vi "MGCC_FntStaMach_Flag_auto.vi"() -> (0 "Array":bool[](array[boolean]))   [LabVIEW 2016]
uses:
  Abnormal Fault State Control/Sub_VIs/Fault_Abnormal_state.vi
  Unplanned islanding (He Yin)/Sub Vis/UnplanISD_Global.vi
panel:
  in  "Feeder #2 energized":bool
  in  "Feeder #1 energized":bool
  in  "PCC_5 IR position":bool
  in  "PCC_4 IR position":bool
  in  "Feeder #5 energized":bool
  in  "Feeder #4 energized":bool
  in  "Feeder #3 energized":bool
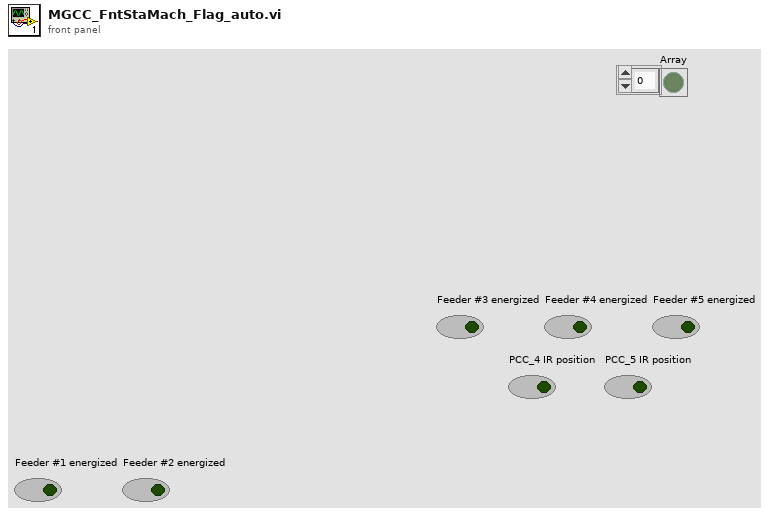
[diagram p1: front panel]
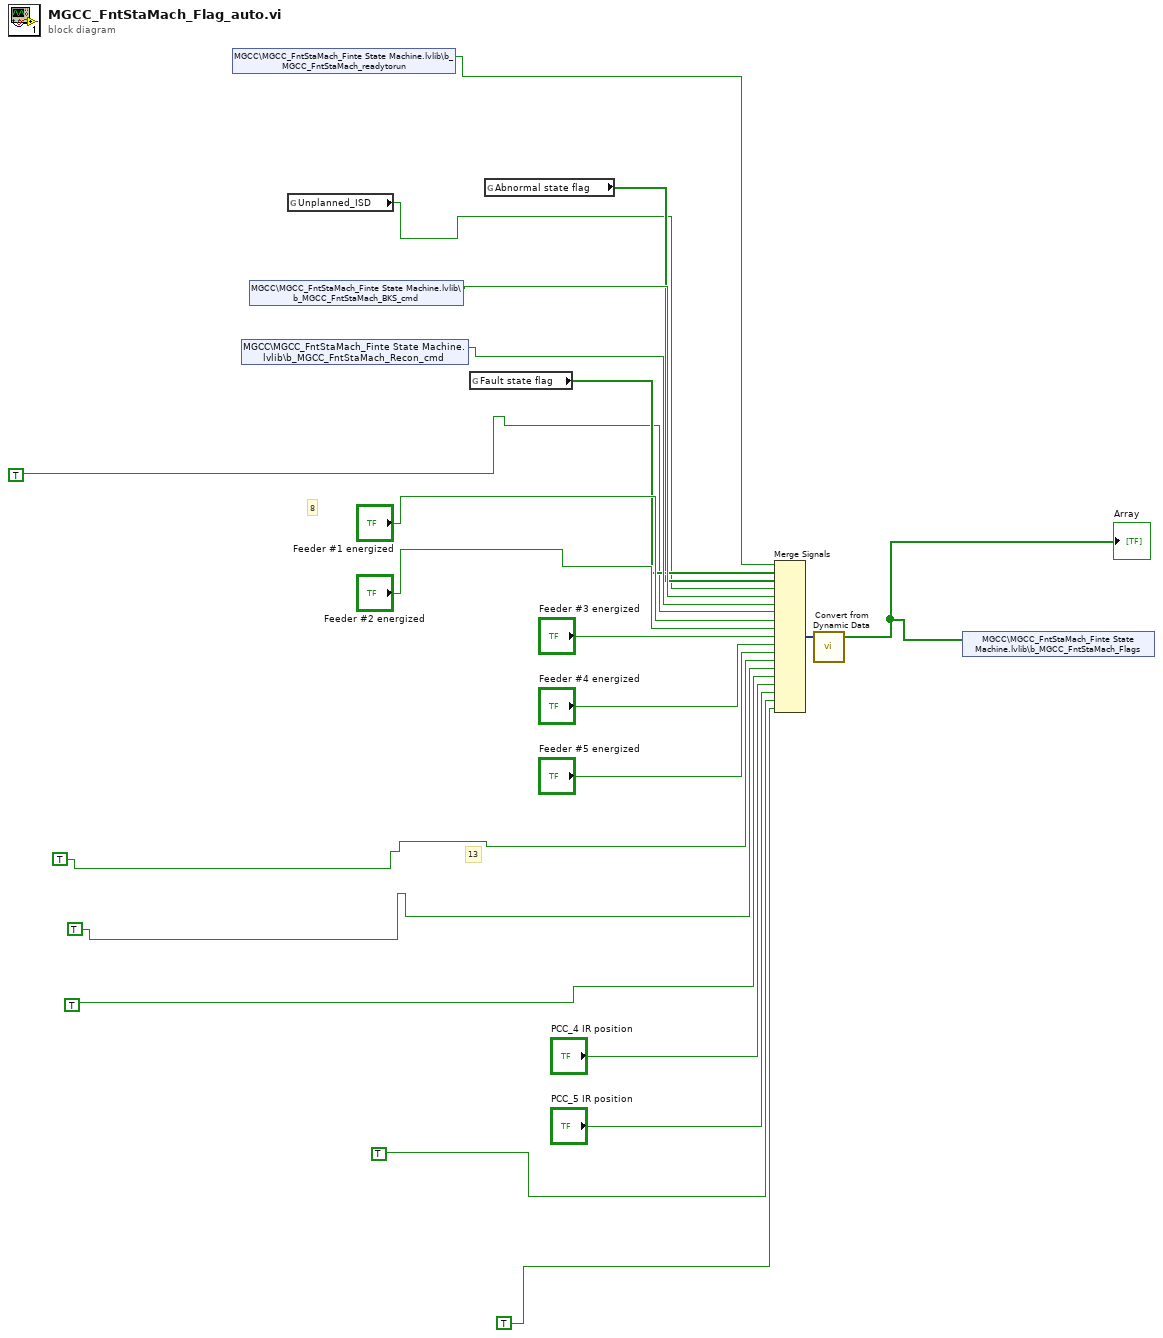
[diagram p0: block diagram]
diagram:
  # "13"
  # "8"
  n1 = shared-variable "MGCC\\MGCC_FntStaMach_Finte State Machine.lvlib\\b_MGCC_FntStaMach_readytorun"() -> (w15:bool)  [unwired: 1 in, 1 out]
  n2 = shared-variable "MGCC\\MGCC_FntStaMach_Finte State Machine.lvlib\\b_MGCC_FntStaMach_Recon_cmd"() -> (w13:bool)  [unwired: 1 in, 1 out]
  n3 = shared-variable "MGCC\\MGCC_FntStaMach_Finte State Machine.lvlib\\b_MGCC_FntStaMach_BKS_cmd"() -> (w14:bool)  [unwired: 1 in, 1 out]
  n4 = global read "UnplanISD_Global.vi" "Unplanned_ISD"() -> (w6:bool)
  n5 = global read "Fault_Abnormal_state.vi" "Fault state flag"() -> (w9:bool[])
  n6 = global read "Fault_Abnormal_state.vi" "Abnormal state flag"() -> (w8:bool[])
  n7 = Merge Signals(w15, w9, w8, w6, w14, w13, TRUE, "Feeder #1 energized", "Feeder #2 energized", "Feeder #3 energized", "Feeder #4 energized", "Feeder #5 energized", TRUE, TRUE, TRUE, "PCC_4 IR position", "PCC_5 IR position", TRUE, TRUE) -> (w21:dynamicdata)
  n8 = call "Convert from Dynamic Data"("Dynamic Data Type"=w21) -> ("Array"=w10:bool[])  [unwired: 3 in]
  "Array" <- w10
  n9 = shared-variable "MGCC\\MGCC_FntStaMach_Finte State Machine.lvlib\\b_MGCC_FntStaMach_Flags"(w10) -> ()  [unwired: 1 in, 1 out]
